vi "Medidor_File.vi"() -> (0 "Corrente Fase C":dynamicdata(graph), 1 "Corrente Fase B":dynamicdata(graph), 2 "Corrente Fase A":dynamicdata(graph), 3 "TimeStamp":dynamicdata(graph), 4 "Tensão Fase C":dynamicdata(graph), 5 "Tensão Fase B":dynamicdata(graph), 6 "Tensão Fase A":dynamicdata(graph))   [LabVIEW 2024]
doc: "Use this template to simulate the acquisition of data by reading data from a file.\nNote: LabVIEW enables automatic error handling by default for VIs you create from this template."
panel:
  out "TimeStamp":string[][](table)
  out "Fase C":string[][](table)
  out "Fase B":string[][](table)
  out "Fase A":string[][](table)
  out "All Data":string[][](table)
  out "Medições":dynamicdata(graph) caption="Waveform Graph"
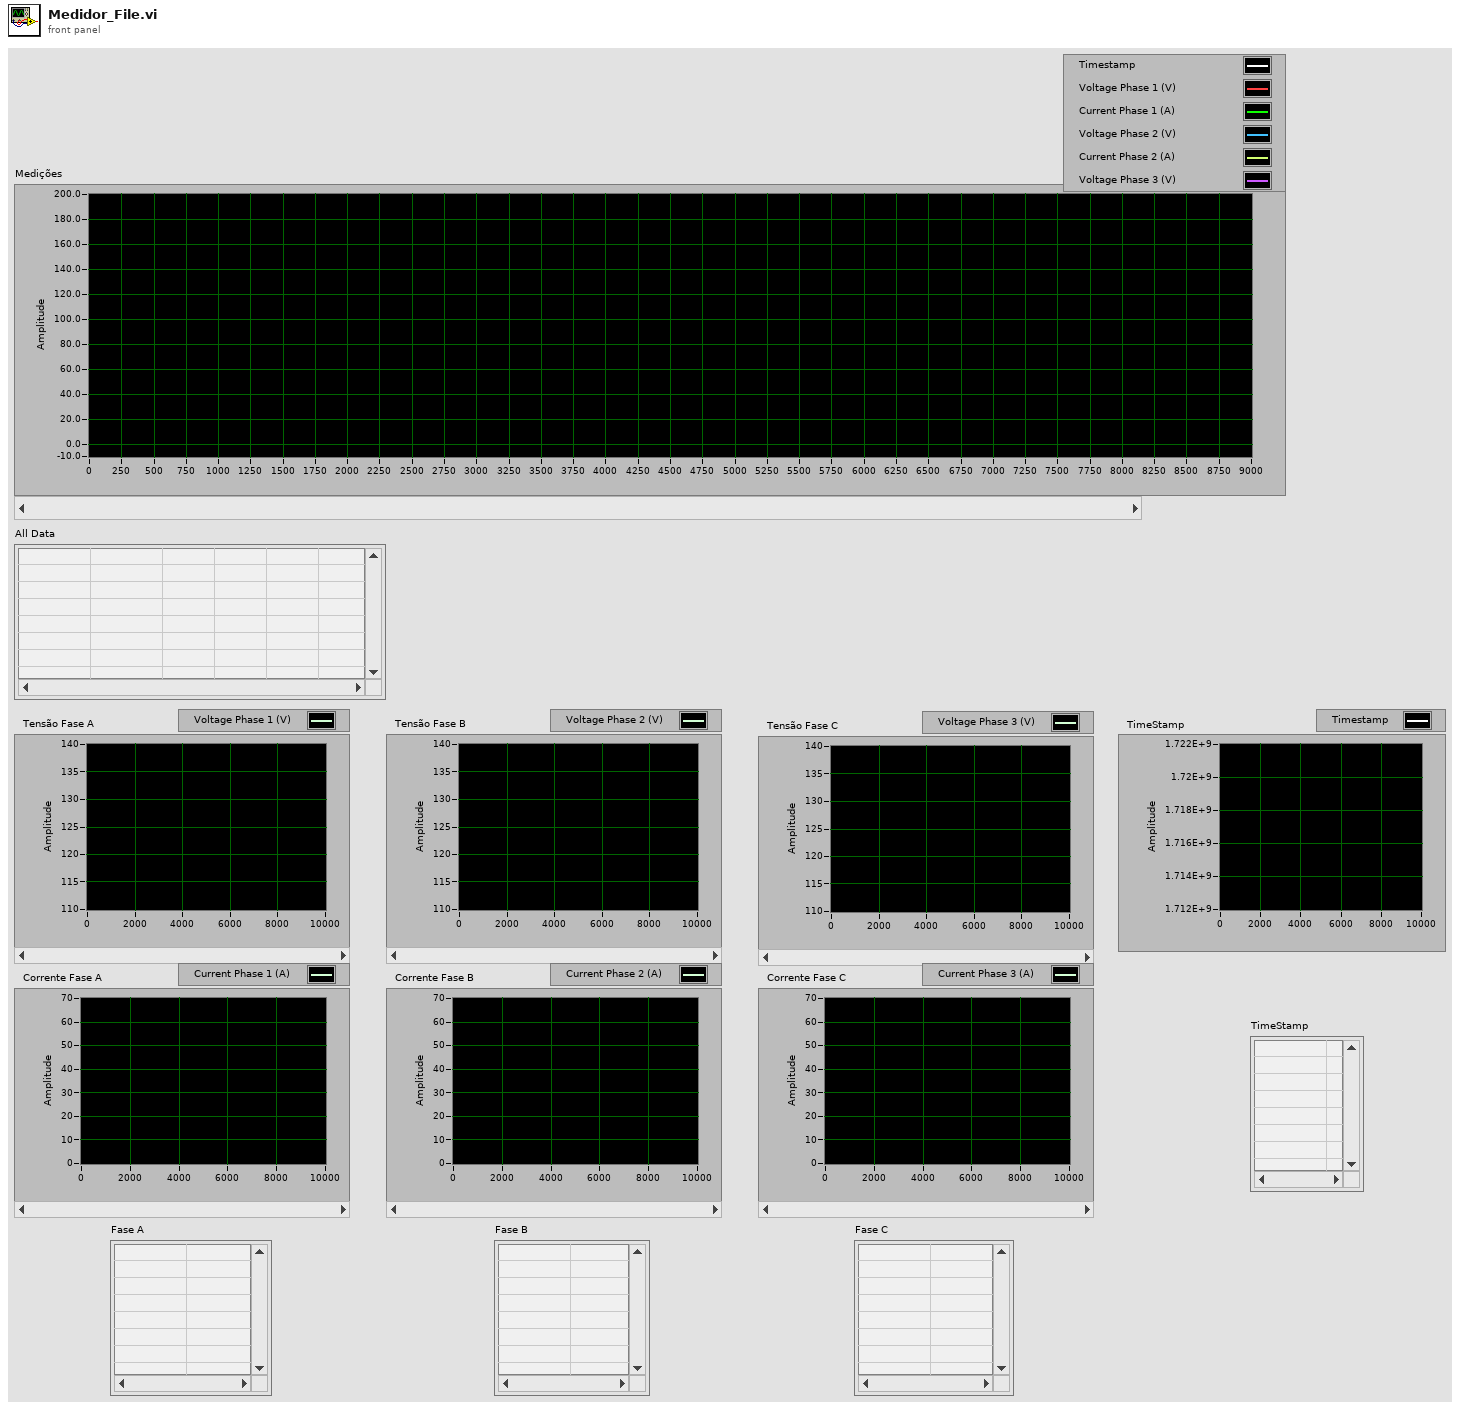
[diagram p1: front panel]
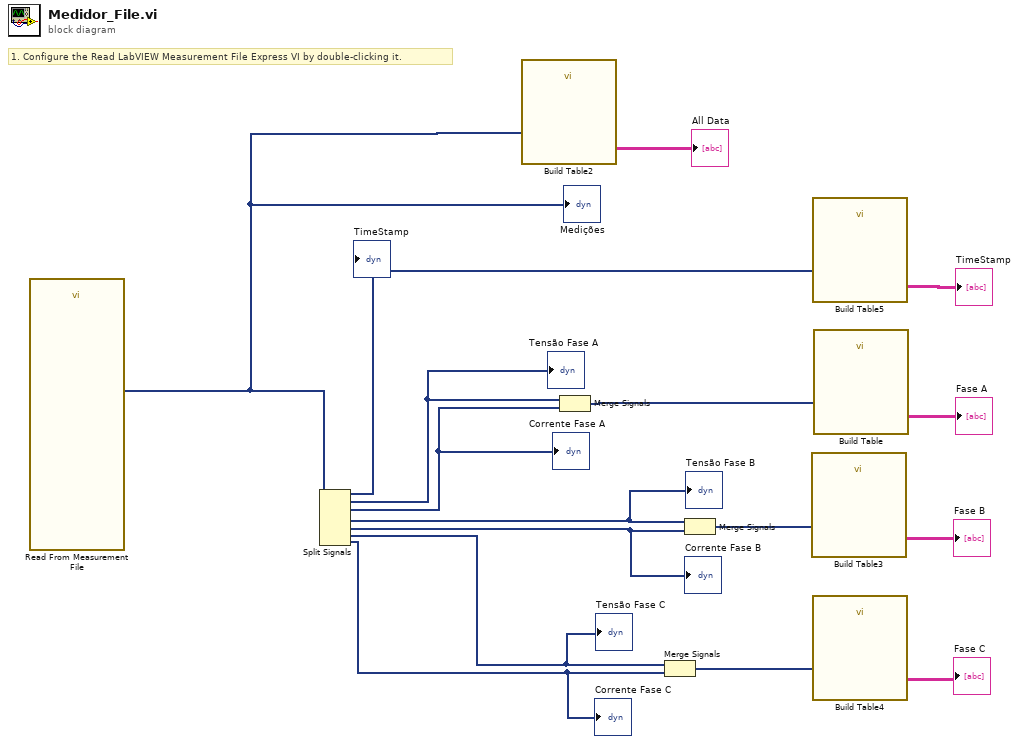
[diagram p0: block diagram]
diagram:
  # "1. Configure the Read LabVIEW Measurement File Express VI by double-clicking it."
  n1 = call "Read From Measurement File"() -> ("Signals"=w10:dynamicdata)  [unwired: 6 in, 5 out]
  "Medições" <- w10
  n2 = Split Signals(w10) -> (w9:dynamicdata, w7:dynamicdata, w6:dynamicdata, w5:dynamicdata, w4:dynamicdata, w1:dynamicdata, w2:dynamicdata)  [unwired: 7 in]
  "TimeStamp" <- w9
  "Tensão Fase A" <- w7
  "Corrente Fase A" <- w6
  "Tensão Fase B" <- w5
  "Corrente Fase B" <- w4
  "Tensão Fase C" <- w1
  "Corrente Fase C" <- w2
  n3 = call "Build Table2"("Signals"=w10) -> ("Table"=→"All Data":string[][])  [unwired: 4 in, 6 out]
  n4 = Merge Signals(w7, w6) -> (w3:dynamicdata)
  n5 = Merge Signals(w1, w2) -> (w11:dynamicdata)
  n6 = Merge Signals(w5, w4) -> (w14:dynamicdata)
  n7 = call "Build Table3"("Signals"=w14) -> ("Table"=→"Fase B":string[][])  [unwired: 4 in, 6 out]
  n8 = call "Build Table5"("Signals"=w9) -> ("Table"=→"TimeStamp":string[][])  [unwired: 4 in, 6 out]
  n9 = call "Build Table4"("Signals"=w11) -> ("Table"=→"Fase C":string[][])  [unwired: 4 in, 6 out]
  n10 = call "Build Table"("Signals"=w3) -> ("Table"=→"Fase A":string[][])  [unwired: 4 in, 6 out]
